vi "Test PLC API.vi"() -> ()   [LabVIEW 2024]
doc: "PLC API Tester."
uses:
  PLC.lvlib
  <vilib>/Utility/error.llb/DialogType.ctl
panel:
  out "Connection Status":map{i32, bool}(c390)
  out "Connection Status":bool
  in  "Connect":bool
  in  "IP":string
  in  "Port":i32
  in  "Set IP":bool
  out "last error":errorcluster
  in  "Show Diagram on Init":bool
  in  "Run as Singleton?":bool
  in  "Show Block Diagram":bool
  in  "Refresh Modules":bool
  out "Active Modules":string[](array[string])
  in  "Stop Module":bool
  in  "Select Module":i32(ring)=-1 caption="Select Module\nTo send Request to" items=["All"=-1]
  in  "Run New Module":bool
  in  "Hide Module Panel":bool
  in  "Show Module Panel":bool
  out "Status":string
  # "This VI tests the API for the Module."
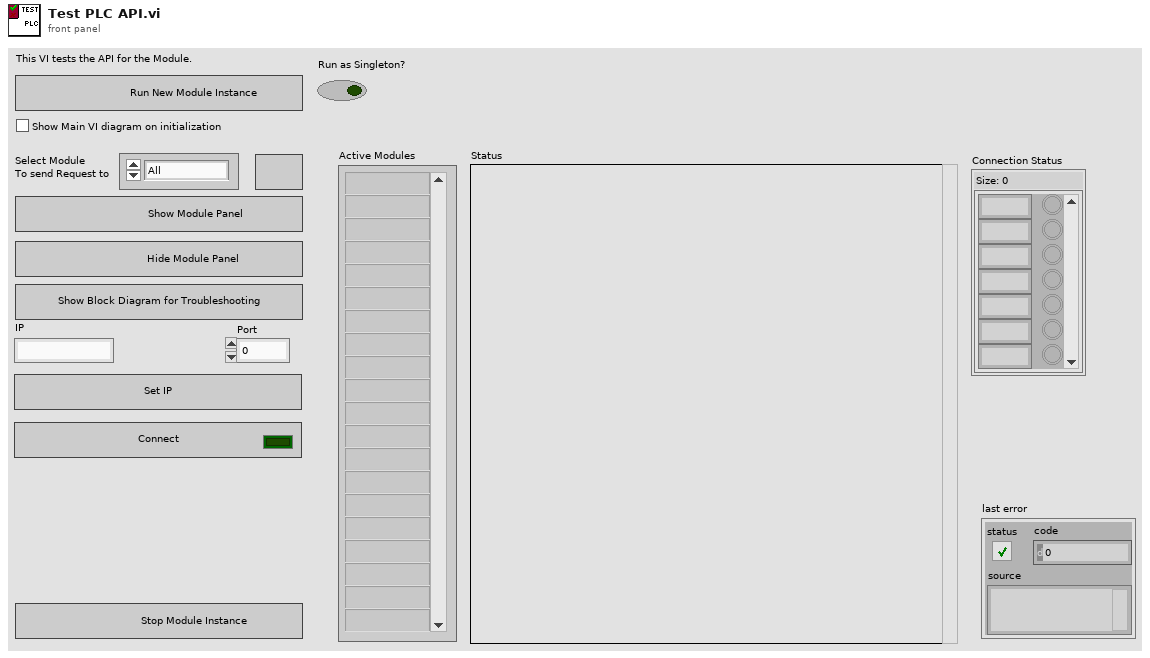
[diagram p1: front panel]
types:
  T1 = typedef "PLC.lvlib/Broadcast Events--cluster.ctl" = cluster{"Module Did Init":refnum<user-event>, "Status Updated":refnum<user-event>, "Error Reported":refnum<user-event>, "Module Did Stop":refnum<user-event>, "Update Module Execution Status":refnum<user-event>, "IP has been Set":refnum<user-event>, "Connection Status Updated":refnum<user-event>}
  T2 = typedef "DialogType.ctl" = u16
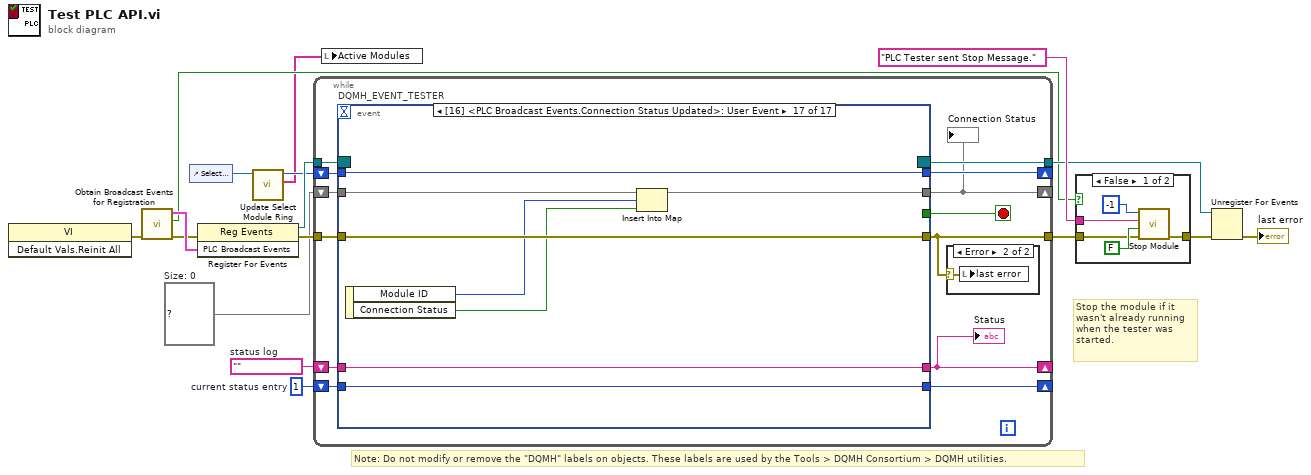
[diagram p0: block diagram]
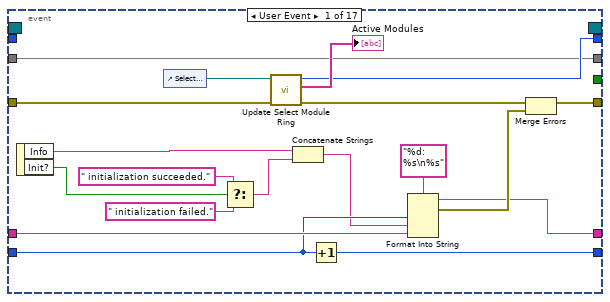
[diagram p4: hidden frame]
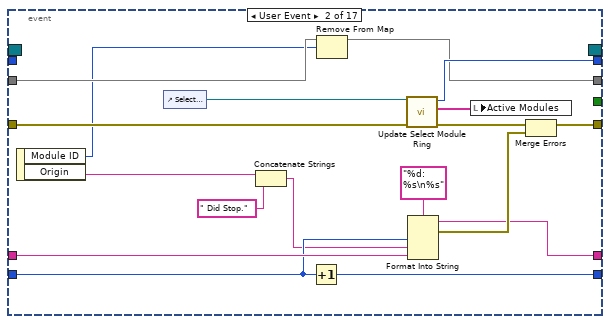
[diagram p5: hidden frame]
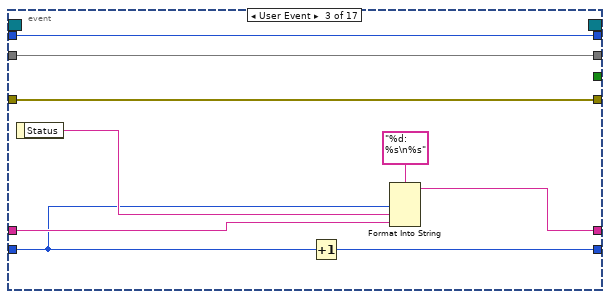
[diagram p6: hidden frame]
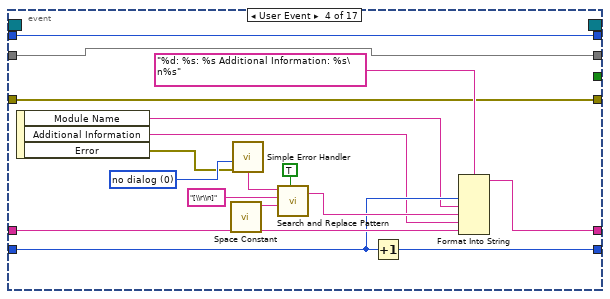
[diagram p7: hidden frame]
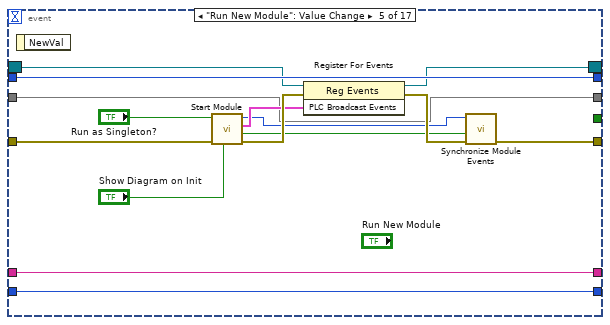
[diagram p8: hidden frame]
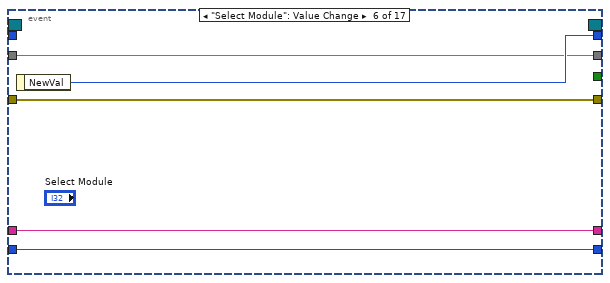
[diagram p9: hidden frame]
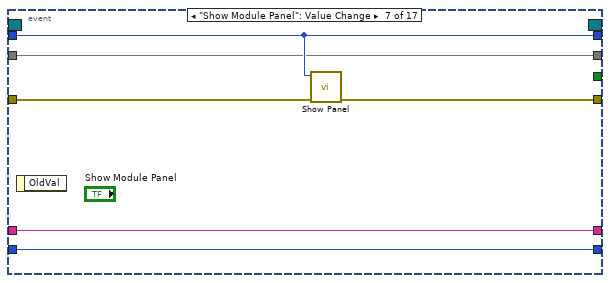
[diagram p10: hidden frame]
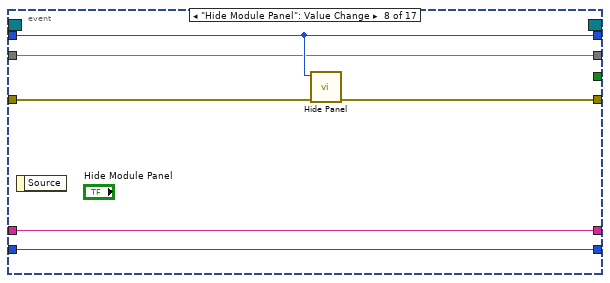
[diagram p11: hidden frame]
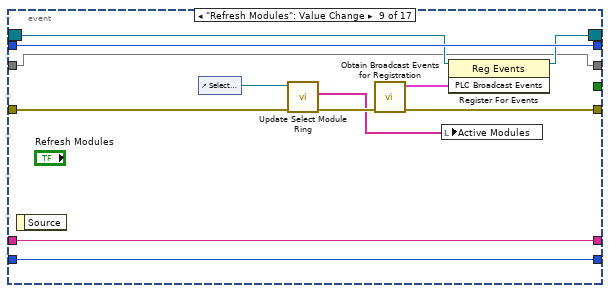
[diagram p12: hidden frame]
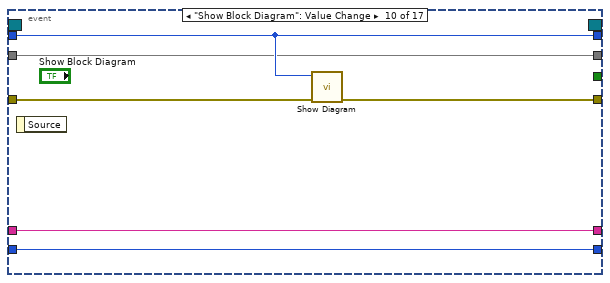
[diagram p13: hidden frame]
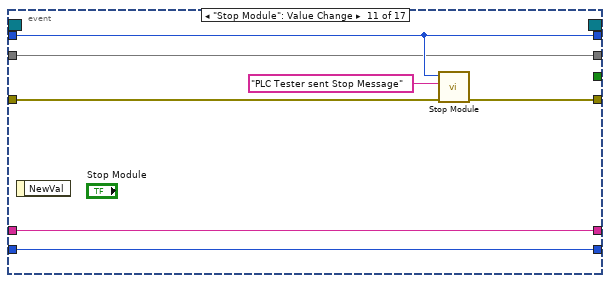
[diagram p14: hidden frame]
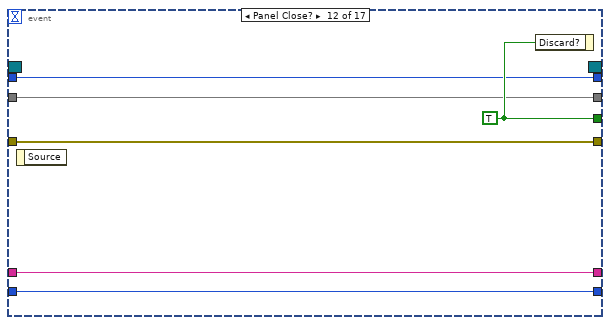
[diagram p15: hidden frame]
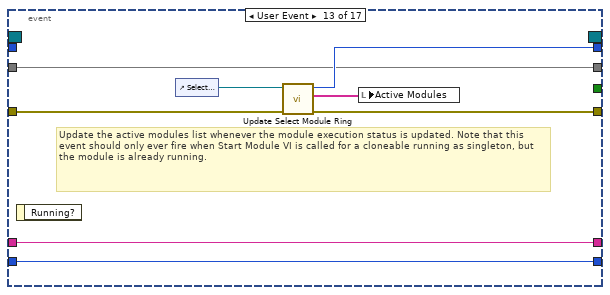
[diagram p16: hidden frame]
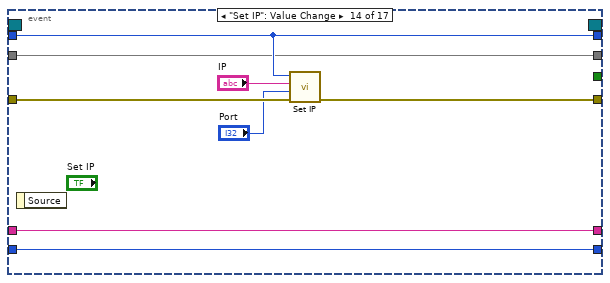
[diagram p17: hidden frame]
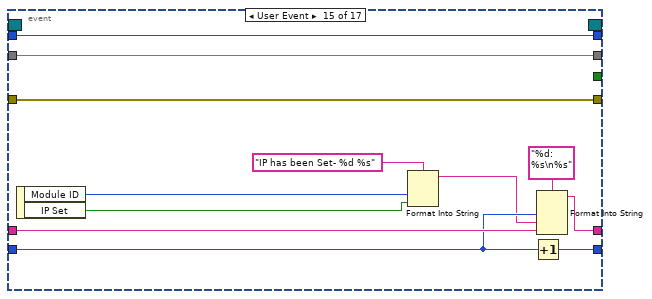
[diagram p18: hidden frame]
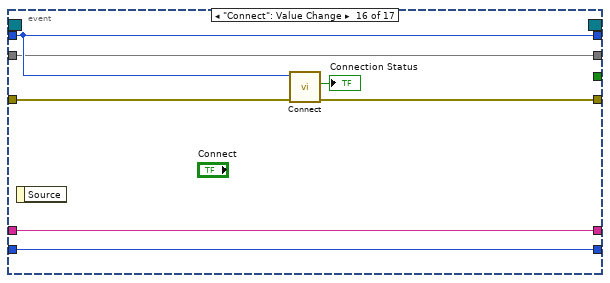
[diagram p19: hidden frame]
diagram:
  w1 = map{i32, bool} {}  # Size: 0
  w14 = 1  # current status entry
  w15 = ""  # status log
  # "Stop the module if it wasn't already running when the tester was started."
  # "Note: Do not modify or remove the \"DQMH\" labels on objects. These labels are used by the Tools > DQMH Consortium > DQMH utilities."
  n1 = invoke class="VI" method="Default Vals.Reinit All"() -> (error out=w9:errorcluster)  [unwired: 3 in, 2 out]
  n2 = call "Obtain Broadcast Events for Registration.vi"("error in"=w9) -> ("error out"=w8:errorcluster, "Already running?"=w7:bool, "PLC Broadcast Events"=w13:T1)  [unwired: 8 in]
  n3 = control-ref of="Select Module"() -> (w4:refnum<vi>)
  n4 = register-events(error in=w8, w13) -> (reference out=w17:refnum<event-registration>, error out=w12:errorcluster)  [unwired: 1 in]
  n5 = call "Update Select Module Ring.vi"("Select Module Ring Ref"=w4) -> ("Active Modules (Array)"=w2:string[], "New Module Ring Value"=w3:i32)  [unwired: 8 in, 1 out]
  n6 = while {
    tunnel: w17 -> [w30]
    tunnel: [w21] -> w6
    tunnel: w12 -> [w29]
    shift-right: [w25] -> _
    shift-left: w15 -> [w27]
    shift-right: [w26] -> _
    shift-left: w14 -> [w28]
    shift-right: [w23] -> _
    shift-left: w3 -> [w24]
    tunnel: [w22] -> w10
    shift-right: [w19] -> _
    shift-left: w1 -> [w18]
    stop <- w20 stop-if-true
    n7 = event "DQMH_EVENT_TESTER" shown="[16] <PLC Broadcast Events.Connection Status Updated>: User Event" {
      selector: w30 -> [_ _ _ _ w103 _ _ _ w133 _ _ _ _ _ _ _ _]
      dyn-events: [_ _ _ _ w102 _ _ _ w132 _ _ _ _ _ _ _ _] -> w22
      timeout: _ -> [_ _ _ _ _ _ _ _ _ _ _ _ _ _ _ _ _]
      tunnel: [_ _ _ _ _ _ _ _ _ _ _ w157 _ _ _ _ _] -> w20
      tunnel: [w40 w60 w77 w82 w101 w114 w119 w125 w129 w141 w147 w156 w161 w169 w185 w188 w200] -> w21
      tunnel: w29 -> [w42 w62 w77 w82 w104 w114 w120 w126 w134 w144 w148 w156 w162 w173 w185 w192 w200]
      tunnel: w28 -> [w47 w65 w70 w85 w106 w112 w117 w123 w137 w142 w150 w154 w164 w171 w181 w190 w197]
      tunnel: w27 -> [w48 w66 w73 w86 w107 w113 w118 w124 w138 w143 w151 w155 w165 w172 w183 w191 w198]
      tunnel: [w45 w63 w74 w84 w107 w113 w118 w124 w138 w143 w151 w155 w165 w172 w182 w191 w198] -> w25
      tunnel: [w46 w64 w76 w83 w106 w112 w117 w123 w137 w142 w150 w154 w164 w171 w180 w190 w197] -> w26
      tunnel: w24 -> [_ _ w71 w94 w105 _ w116 w122 w136 w140 w149 w153 _ w170 w184 w189 w199]
      tunnel: [w37 w57 w71 w94 w105 w111 w116 w122 w136 w140 w149 w153 w160 w170 w184 w189 w199] -> w23
      tunnel: [w32 w51 w69 w78 w95 w110 w115 w121 w127 w139 w145 w152 w158 w166 w174 w186 w194] -> w19
      tunnel: w18 -> [w32 w53 w69 w78 w95 w110 w115 w121 w127 w139 w145 w152 w158 w166 w174 w186 w193]
      event User Event {
        n8 = event-data() -> ("Info"=w44:string, "Init?"=w34:bool)  [unwired: 1 in]
        n9 = control-ref of="Select Module"() -> (w39:refnum<vi>)
        n10 = Select(t=" initialization succeeded.", s=w34, f=" initialization failed.") -> (s? t:f=w33:string)
        n11 = call "Update Select Module Ring.vi"("error in"=w42, "Select Module Ring Ref"=w39) -> ("error out"=w41:errorcluster, "Active Modules (Array)"=→"Active Modules":string[], "New Module Ring Value"=w37:i32)  [unwired: 7 in]
        n12 = Concatenate Strings(w44, w33) -> (w43:string)
        n13 = Increment(x=w47) -> (x+1=w46:i32)
        n14 = Format Into String(format string="%d: %s\n%s", w47, w43, w48) -> (resulting string=w45:string, error out=w50:errorcluster)  [unwired: 2 in]
        n15 = Merge Errors(w41, w50) -> (w40:errorcluster)
      }
      event User Event {
        n16 = event-data() -> ("Module ID"=w52:i32, "Origin"=w55:string)  [unwired: 1 in]
        n17 = control-ref of="Select Module"() -> (w59:refnum<vi>)
        n18 = Concatenate Strings(w55, " Did Stop.") -> (w54:string)
        n19 = Increment(x=w65) -> (x+1=w64:i32)
        n20 = Remove From Map(10:w52, 11:w53) -> (3:w51:map{i32, bool})  [unwired: 2 out]
        n21 = call "Update Select Module Ring.vi"("error in"=w62, "Select Module Ring Ref"=w59) -> ("error out"=w61:errorcluster, "Active Modules (Array)"=w58:string[], "New Module Ring Value"=w57:i32)  [unwired: 7 in]
        n22 = Format Into String(format string="%d: %s\n%s", w65, w54, w66) -> (resulting string=w63:string, error out=w68:errorcluster)  [unwired: 2 in]
        n23 = local write "Active Modules"(w58) -> ()
        n24 = Merge Errors(w61, w68) -> (w60:errorcluster)
      }
      event User Event {
        n25 = event-data() -> ("Status"=w72:string)  [unwired: 1 in]
        n26 = Increment(x=w70) -> (x+1=w76:i32)
        n27 = Format Into String(format string="%d: %s\n%s", w70, w72, w73) -> (resulting string=w74:string)  [unwired: 2 in, 1 out]
      }
      event User Event {
        w87 = T2 0 items=["no dialog", "OK message", "continue or stop message", "OK message + warnings", "continue/stop + warnings"] ("type of dialog (OK msg:1)")
        n28 = event-data() -> ("Module Name"=w81:string, "Additional Information"=w80:string, "Error"=w79:errorcluster)  [unwired: 1 in]
        n29 = call <vilib>:"Space Constant.vi"() -> ("String"=w91:string)
        n30 = call <vilib>:"Simple Error Handler.vi"("type of dialog (OK msg:1)"=w87, "error in (no error)"=w79) -> ("message"=w88:string)  [unwired: 3 in, 4 out]
        n31 = call <vilib>:"Search and Replace Pattern.vi"("string"=w88, "regular expression (\"\")"="[\\r\\n]" ("regular expression (\"\")"), "replace string (\"\")"=w91, "replace all? (F)"=TRUE ("replace all CR/LF with spaces")) -> ("result string"=w89:string)  [unwired: 1 in, 1 out]
        n32 = Increment(x=w85) -> (x+1=w83:i32)
        n33 = Format Into String(format string="%d: %s: %s Additional Information: %s\n%s", w85, w81, w89, w80, w86) -> (resulting string=w84:string)  [unwired: 2 in, 1 out]
      }
      event "Run New Module": Value Change {
        n34 = event-data() -> ()  [unwired: 1 in, 1 out]
        n35 = call "Start Module.vi"("Show Main VI Diagram on Init (F)"="Show Diagram on Init", "error in"=w104, "Run as Singleton? (F)"="Run as Singleton?") -> ("error out"=w108:errorcluster, "Wait for Event Sync?"=w100:bool, "PLC Broadcast Events"=w99:T1, "Module ID"=w96:i32)  [unwired: 4 in, 1 out]
        n36 = register-events(reference=w103, error in=w108, w99) -> (reference out=w102:refnum<event-registration>, error out=w109:errorcluster)
        n37 = call "Synchronize Module Events.vi"("error in"=w109, "Wait for Event Sync?"=w100, "Module ID in"=w96) -> ("error out"=w101:errorcluster)  [unwired: 7 in, 1 out]
      }
      event "Select Module": Value Change {
        n38 = event-data() -> ("NewVal"=w111:i32)  [unwired: 1 in]
      }
      event "Show Module Panel": Value Change {
        n39 = event-data() -> ()  [unwired: 1 in, 1 out]
        n40 = call "Show Panel.vi"("error in"=w120, "Module ID"=w116) -> ("error out"=w119:errorcluster)  [unwired: 9 in]
      }
      event "Hide Module Panel": Value Change {
        n41 = event-data() -> ()  [unwired: 1 in, 1 out]
        n42 = call "Hide Panel.vi"("error in"=w126, "Module ID"=w122) -> ("error out"=w125:errorcluster)  [unwired: 9 in]
      }
      event "Refresh Modules": Value Change {
        n43 = event-data() -> ()  [unwired: 1 in, 1 out]
        n44 = control-ref of="Select Module"() -> (w135:refnum<vi>)
        n45 = call "Update Select Module Ring.vi"("error in"=w134, "Select Module Ring Ref"=w135) -> ("error out"=w130:errorcluster, "Active Modules (Array)"=w128:string[])  [unwired: 7 in, 1 out]
        n46 = call "Obtain Broadcast Events for Registration.vi"("error in"=w130) -> ("error out"=w129:errorcluster, "PLC Broadcast Events"=w131:T1)  [unwired: 8 in, 1 out]
        n47 = local write "Active Modules"(w128) -> ()
        n48 = register-events(reference=w133, w131) -> (reference out=w132:refnum<event-registration>)  [unwired: 1 in, 1 out]
      }
      event "Show Block Diagram": Value Change {
        n49 = event-data() -> ()  [unwired: 1 in, 1 out]
        n50 = call "Show Diagram.vi"("error in"=w144, "Module ID"=w140) -> ("error out"=w141:errorcluster)  [unwired: 9 in]
      }
      event "Stop Module": Value Change {
        n51 = event-data() -> ()  [unwired: 1 in, 1 out]
        n52 = call "Stop Module.vi"("error in"=w148, "Origin"="PLC Tester sent Stop Message", "Module ID"=w149) -> ("error out"=w147:errorcluster)  [unwired: 8 in]
      }
      event Panel Close? {
        w157 = TRUE ("Discard?")
        n53 = event-data() -> ()  [unwired: 1 in, 1 out]
        n54 = event-data("Discard?"=w157) -> ()  [unwired: 1 in, 1 out]
      }
      event User Event {
        # "Update the active modules list whenever the module execution status is updated. Note that this event should only ever fire when Start Module VI is called for a cloneable running as singleton, but the module is already running."
        n55 = event-data() -> ()  [unwired: 1 in, 1 out]
        n56 = control-ref of="Select Module"() -> (w163:refnum<vi>)
        n57 = call "Update Select Module Ring.vi"("error in"=w162, "Select Module Ring Ref"=w163) -> ("error out"=w161:errorcluster, "Active Modules (Array)"=w159:string[], "New Module Ring Value"=w160:i32)  [unwired: 7 in]
        n58 = local write "Active Modules"(w159) -> ()
      }
      event "Set IP": Value Change {
        n59 = event-data() -> ()  [unwired: 1 in, 1 out]
        n60 = call "Set IP.vi"("error in"=w173, "Port"="Port", "IP"="IP", "Module ID"=w170) -> ("error out"=w169:errorcluster)  [unwired: 7 in]
      }
      event User Event {
        n61 = event-data() -> ("Module ID"=w176:i32, "IP Set"=w175:bool)  [unwired: 1 in]
        n62 = Format Into String(format string="IP has been Set- %d %s", w176, w175) -> (resulting string=w177:string)  [unwired: 2 in, 1 out]
        n63 = Increment(x=w181) -> (x+1=w180:i32)
        n64 = Format Into String(format string="%d: %s\n%s", w181, w177, w183) -> (resulting string=w182:string)  [unwired: 2 in, 1 out]
      }
      event "Connect": Value Change {
        n65 = event-data() -> ()  [unwired: 1 in, 1 out]
        n66 = call "Connect.vi"("error in"=w192, "Module ID"=w189) -> ("error out"=w188:errorcluster, "Connection Status"=→"Connection Status":bool)  [unwired: 7 in, 1 out]
      }
      event User Event {
        n67 = event-data() -> ("Module ID"=w196:i32, "Connection Status"=w195:bool)  [unwired: 1 in]
        n68 = Insert Into Map(map in=w193, key=w196, value=w195) -> (map out=w194:map{i32, bool})  [unwired: 2 out]
      }
    }
    "Status" <- w25
    "Connection Status" <- w19
    n69 = case shown="Error" w21 {
      selector: w21 -> [_ w31]
      frame No Error {
      }
      frame Error {
        n70 = local write "last error"(w31) -> ()
      }
    }
  }
  n71 = local write "Active Modules"(w2) -> ()
  n72 = case shown="False" w7 {
    tunnel: [w205 w206] -> w16
    tunnel: "PLC Tester sent Stop Message." ("Origin") -> [w204 _]
    tunnel: w6 -> [w201 w206]
    frame False {
      n73 = call "Stop Module.vi"("error in"=w201, "Wait for Module to stop? (F)"=FALSE ("Wait for Module to stop?"), "Origin"=w204, "Module ID"=-1 ("Stop all")) -> ("error out"=w205:errorcluster)  [unwired: 7 in]
    }
    frame True {
    }
  }
  n74 = Unregister For Events(event registration refnum=w10, error in=w16) -> (error out=→"last error":errorcluster)
